vi "Set Splitter Size.vi"(8 "error in (no error)":errorcluster, 10 "Splitter size [2]":i32=2, 11 "Divider in":refnum<class "Divider.lvclass">) -> (0 "error out":errorcluster, 3 "Divider out":refnum<class "Divider.lvclass">)   [LabVIEW 2021, in "Divider.lvclass"]
doc: "Copyright 2018, Wiebe Walstra, wiebe@carya.nl."
uses:
  Divider.lvclass
  Divider.lvclass/Divider.ctl
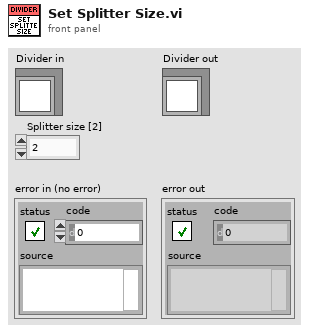
[diagram p1: front panel]
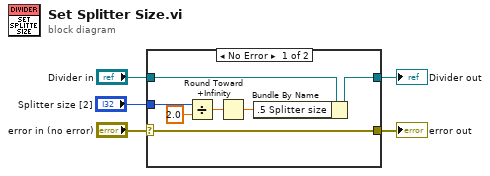
[diagram p0: block diagram]
diagram:
  n1 = case shown="No Error" "error in (no error)" {
    selector: "error in (no error)" -> [w12 w14]
    tunnel: [w12 w14] -> w4
    tunnel: [w7 w13] -> w2
    tunnel: "Divider in" -> [w8 w13]
    tunnel: "Splitter size [2]" -> [w6 _]
    frame No Error {
      n2 = Divide(x=w6, y=2.0) -> (x/y=w11:dbl)
      n3 = Round Toward +Infinity(x=w11) -> (ceil(x): smallest int >= x=w9:dbl)
      n4 = Bundle By Name(cluster=w8, ".5 Splitter size"=w9) -> (w7:refnum<class "Divider.lvclass">)
    }
    frame Error {
    }
  }
  "error out" <- w4
  "Divider out" <- w2
